vi "Select Config.vi"(7 "String":string="Launcher", 8 "error in (no error)":errorcluster, 10 "item tag":string, 11 "menu reference":refnum<k9>) -> (0 "error out":errorcluster)   [LabVIEW 2025, in "Full User Interface.lvlib"]
uses:
  Full User Interface.lvlib
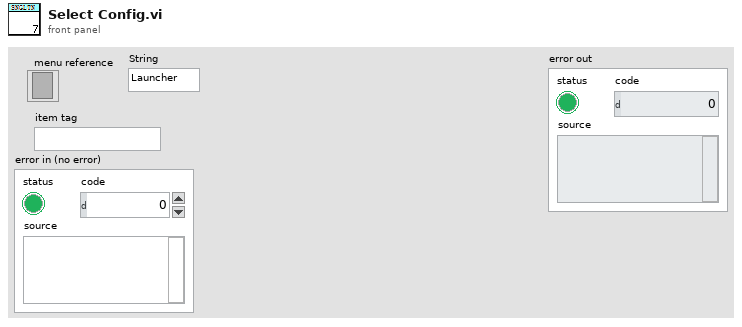
[diagram p1: front panel]
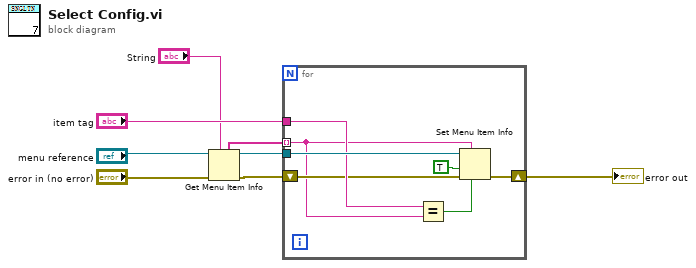
[diagram p0: block diagram]
diagram:
  n1 = Get Menu Item Info(7:"String", 8:"error in (no error)", 11:"menu reference") -> (0:w3:errorcluster, 3:w5:refnum<k9>, 5:w4:string[])  [unwired: 4 out]
  n2 = for {
    tunnel: "item tag" -> [w14]
    tunnel: w5 -> [w15]
    tunnel: w4 -> [w11] mode=indexing
    shift-right: [w13] -> w2
    shift-left: w3 -> [w12]
    n3 = Equal?(x=w14, y=w11) -> (x = y?=w9:bool)
    n4 = Set Menu Item Info(6:w9, 7:w11, 8:w12, 9:TRUE ("enabled"), 11:w15) -> (0:w13:errorcluster)  [unwired: 2 in, 1 out]
  }
  "error out" <- w2
